vi "onStop.vi"(8 "error in (no error)":errorcluster, 11 "Inst.Transport":refnum<class "Inst.Transport.lvclass">) -> (0 "error out":errorcluster, 3 "Inst.Transport out":refnum<class "Inst.Transport.lvclass">)   [LabVIEW 2019, in "Inst.Transport.lvclass"]
uses:
  Inst.Transport.lvclass
  Inst.Transport.lvclass/Inst.Transport.ctl
  <userlib>/LevyLab/Instrument Framework/Instrument Types/SCPI/Instrument.SCPI.lvclass
  Transport/Transport.lvclass
panel:
  # "For instructions on how to use the JKI State Machine Objects, examples and video tutorials, visit:\nhttp://jki.net/state-machine-objects/\n\nJKI State Machine Objects™\nhttp://jki.net/state-machine-objects/\nCopyright (C) 2005-2015, JKI <info@jki.net>\nALL RIGHTS RESERVED"
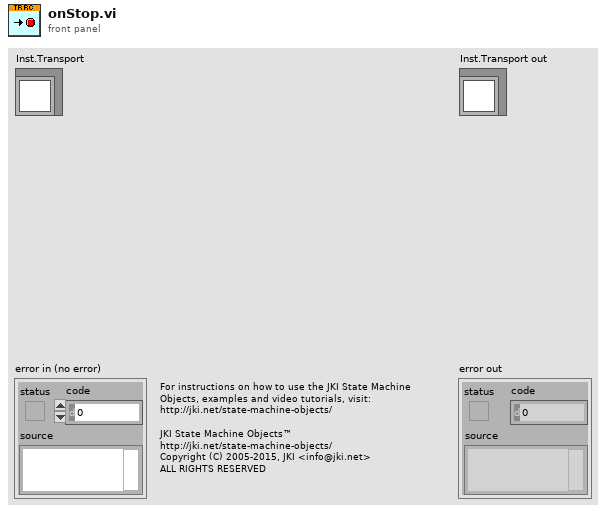
[diagram p1: front panel]
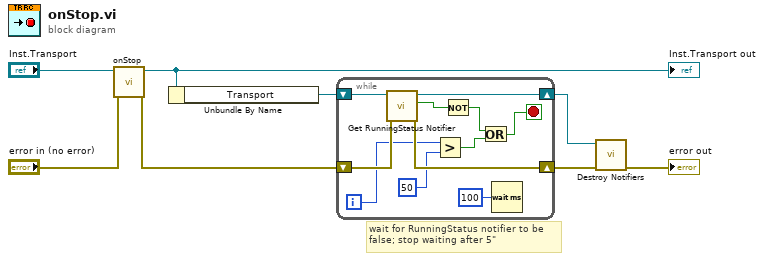
[diagram p0: block diagram]
diagram:
  # "wait for RunningStatus notifier to be\nfalse; stop waiting after 5\""
  n1 = call-parent "onStop.vi"("error in (no error)"="error in (no error)", "SMO"="Inst.Transport") -> ("error out"=w4:errorcluster, "SMO out"=w5:refnum<class "Inst.Transport.lvclass">)  [unwired: 8 in]
  "Inst.Transport out" <- w5
  n2 = Unbundle By Name(w5) -> ("Transport"=w2:refnum<class "Transport.lvclass">)
  n3 = while {
    shift-right: [w18] -> w3
    shift-left: w4 -> [w19]
    shift-right: [w16] -> w1
    shift-left: w2 -> [w17]
    i -> [w10]
    stop <- w13 stop-if-true
    n4 = call "Get RunningStatus Notifier.vi"("error in (no error)"=w19, "Transport in"=w17) -> ("error out"=w18:errorcluster, "Running?"=w12:bool, "Transport out"=w16:refnum<class "Transport.lvclass">)  [unwired: 7 in]
    n5 = Greater?(x=w10, y=50) -> (0:w14:bool)
    n6 = Not(x=w12) -> (.not. x?=w11:bool)
    n7 = Or(x=w11, y=w14) -> (x .or. y?=w13:bool)
    n8 = Wait (ms)(milliseconds to wait=u32 100) -> ()  [unwired: 1 out]
  }
  n9 = call "Destroy Notifiers.vi"("error in (no error)"=w3, "Transport in"=w1) -> ("error out"=→"error out":errorcluster)  [unwired: 9 in]
